vi "send_receive.vi"(7 "Number of try":i32=1, 8 "error in (no error)":errorcluster, 9 "time":u32, 10 "data in":string, 11 "connection ID in":refnum<k5>) -> (0 "error out":errorcluster, 1 "Result":bool, 2 "data out":string, 3 "connection ID out":refnum<k5>)   [LabVIEW 2017]
panel:
  in  "mode":T1(ring)=enum."CRLF"
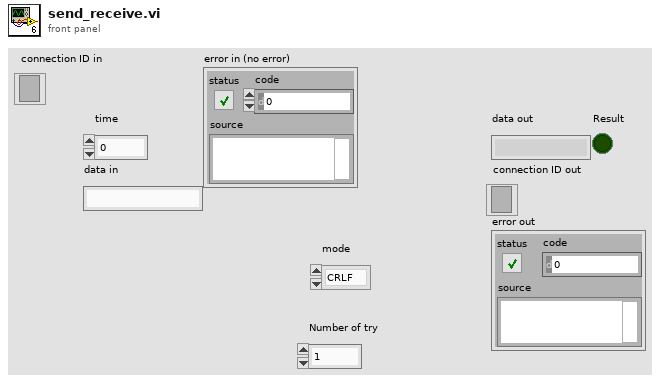
[diagram p1: front panel]
types:
  T1 = enum16{"Standard", "Buffered", "CRLF", "Immediate"}
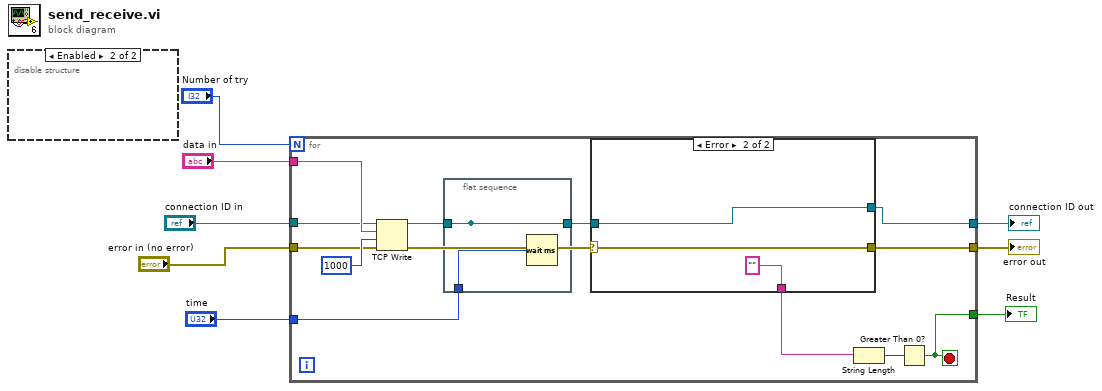
[diagram p0: block diagram]
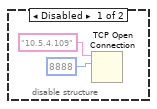
[diagram p2: hidden frame]
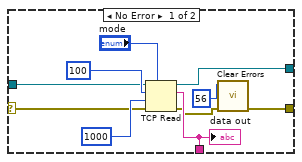
[diagram p3: hidden frame]
diagram:
  n1 = disable-structure shown="Enabled" {
    frame Disabled {
      n2 = TCP Open Connection(address="10.5.4.109", remote port or service name=u16 8888) -> ()  [unwired: 3 in, 2 out]
    }
    frame Enabled {
    }
  }
  n3 = for {
    N: "Number of try" -> [_]
    tunnel: "time" -> [w19]
    tunnel: "data in" -> [w18]
    tunnel: [w14] -> w4
    tunnel: [w13] -> w3
    tunnel: [w20] -> w8
    tunnel: "error in (no error)" -> [w12]
    tunnel: "connection ID in" -> [w11]
    stop <- w14 stop-if-true
    n4 = TCP Write(connection ID=w11, data in=w18, error in (no error)=w12, 9:1000 ("timeout ms (25000)")) -> (connection ID out=w23:refnum<k5>, error out=w21:errorcluster)  [unwired: 1 out]
    n5 = flat-sequence {
      tunnel: w23 -> [w37]
      tunnel: [w37] -> _
      tunnel: w19 -> [w38]
      tunnel: [w37] -> w17
      frame #0 {
        n6 = Wait (ms)(milliseconds to wait=w38) -> ()  [unwired: 1 out]
      }
    }
    n7 = case shown="Error" w21 {
      selector: w21 -> [w29 w35]
      tunnel: w17 -> [w31 w36]
      tunnel: [w25 w35] -> w13
      tunnel: [w30 w36] -> w20
      tunnel: [w28 "" ("data out")] -> w15
      frame No Error {
        n8 = TCP Read(connection ID=w31, bytes to read=100, error in (no error)=w29, 7:"mode", 9:1000 ("timeout ms (25000)")) -> (connection ID out=w30:refnum<k5>, data out=w28:string, error out=w26:errorcluster)
        "data out" <- w28
        n9 = call <vilib>:"Clear Errors.vi"("error in (no error)"=w26, "specific error code to clear (0: all)"=56) -> ("error out"=w25:errorcluster)  [unwired: 4 in, 1 out]
      }
      frame Error {
      }
    }
    n10 = String Length(string=w15) -> (length=w16:i32)
    n11 = Greater Than 0?(x=w16) -> (x > 0?=w14:bool)
  }
  "connection ID out" <- w8
  "error out" <- w3
  "Result" <- w4
